vi "Log to PGSQL subVI.vi"(8 "error in (no error)":errorcluster, 10 "Data":variant, 11 "paths":string) -> (0 "error out":errorcluster)   [LabVIEW 2016]
uses:
  <userlib>/LevyLab/postgreSQL-timescaleDB/Data.PG/Data.PGSQL.lvclass
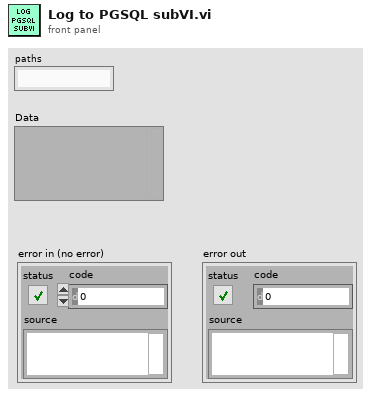
[diagram p1: front panel]
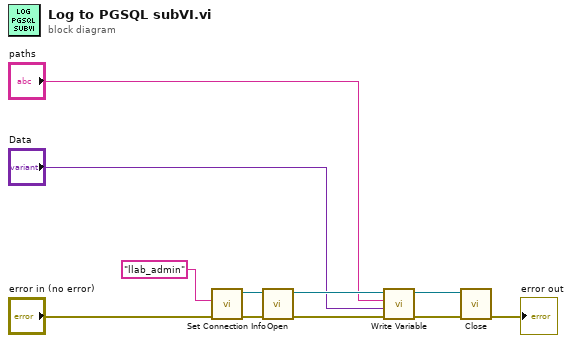
[diagram p0: block diagram]
diagram:
  n1 = call <userlib>:"Set Connection Info.vi"("username"="llab_admin", "error in (no error)"="error in (no error)") -> ("Data.PG out"=w8:refnum<class "Data.PGSQL.lvclass">, "error out"=w7:errorcluster)  [unwired: 7 in]
  n2 = call-dynamic "Open.vi"("error in (no error)"=w7, "Data.PG in"=w8) -> ("error out"=w10:errorcluster, "Data.PG out"=w9:refnum<class "Data.PGSQL.lvclass">)  [unwired: 8 in]
  n3 = call <userlib>:"Write Variable.vi"("error in (no error)"=w10, "Data"="Data", "variable"="paths", "Data.PG in"=w9) -> ("error out"=w3:errorcluster, "Data.PG out"=w4:refnum<class "Data.PGSQL.lvclass">)  [unwired: 5 in, 1 out]
  n4 = call-dynamic "Close.vi"("error in (no error)"=w3, "Data.PG in"=w4) -> ("error out"=→"error out":errorcluster)  [unwired: 8 in, 1 out]
